vi "RollerProcessInput.vi"(5 "OffState":T1, 7 "ReverseState":T1, 8 "error in":errorcluster, 9 "Backward?":bool, 10 "Forward?":bool, 11 "ForwardState":T1) -> (0 "error out":errorcluster, 2 "StateOut":T1)   [LabVIEW 2013]
uses:
  <vilib>/Rock Robotics/WPI/Relay/WPI_RelayValue.ctl
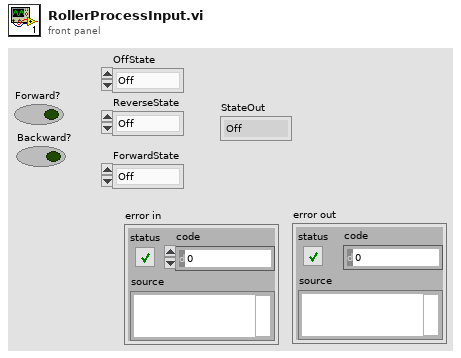
[diagram p1: front panel]
types:
  T1 = typedef "WPI_RelayValue.ctl" = enum16{"Off", "On", "Forward", "Reverse"}
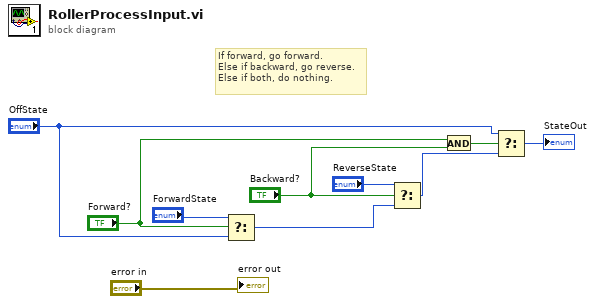
[diagram p0: block diagram]
diagram:
  # "If forward, go forward.\nElse if backward, go reverse.\nElse if both, do nothing."
  n1 = Select(t="ForwardState", s="Forward?", f="OffState") -> (s? t:f=w6:T1)
  n2 = Select(t="ReverseState", s="Backward?", f=w6) -> (s? t:f=w10:T1)
  n3 = And(x="Forward?", y="Backward?") -> (x .and. y?=w9:bool)
  n4 = Select(t="OffState", s=w9, f=w10) -> (s? t:f=→"StateOut":T1)
  "error out" <- "error in"
